vi "Teleop.vi"(10 "Match Info":T1={"Autonomous Elapsed Seconds"=0.0, "TeleOp Elapsed Seconds"=0.0, "Disabled Elapsed Seconds"=0.0, "Visited Autonomous"=FALSE, "Visited TeleOp"=FALSE, "Visited Disabled"=FALSE, "Autonomous Settings"={"Autonomous Style"=enum."Independent", "VI Refnum"=refnum}}, 11 "Call Context":T2) -> ()   [LabVIEW 2015]
doc: "This VI is called for each TeleOp packet received from the DS where the robot is not disabled. It is often used to read from the joysticks and update I/O or to update setpoints for timed control loops. It should complete and return within 20 milliseconds or it may miss DS packets."
uses:
  <vilib>/Rock Robotics/WPI/DriverStation/WPI_DriverStationDerivedRobotMode.ctl
  <vilib>/Rock Robotics/WPI/DriverStation/WPI_DriverStationMatch Info.ctl
  Refname/Refname Enum (Joystick).ctl
  Typedefs/Logitech Axis Mapping.ctl
  Action/Action Name.ctl
  Refname/Refname to String (Joystick).vi
  <vilib>/Rock Robotics/WPI/Utilities/WPI_GetSetVariantRefNum.vi
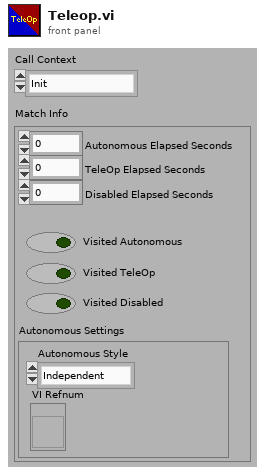
[diagram p1: front panel]
types:
  T1 = typedef "WPI_DriverStationMatch Info.ctl" = cluster{"Autonomous Elapsed Seconds":dbl, "TeleOp Elapsed Seconds":dbl, "Disabled Elapsed Seconds":dbl, "Visited Autonomous":bool, "Visited TeleOp":bool, "Visited Disabled":bool, "Autonomous Settings":cluster{"Autonomous Style":enum16{"Iterative", "Independent"}, "VI Refnum":refnum<vi>}}
  T2 = typedef "WPI_DriverStationDerivedRobotMode.ctl" = enum16{"Init", "Execute", "Stop"}
  T3 = typedef "Refname Enum (Joystick).ctl" = enum16{"Joystick 0", "Joystick 1", "Joystick 2", "Joystick 3"}
  T4 = typedef "WPI_JoystickDevRef.ctl" = cluster{"Device":T5}
  T5 = typedef "WPI_JoystickDeviceEnum.ctl" = enum16{"USB 0", "USB 1", "USB 2", "USB 3", "USB 4", "USB 5"}
  T6 = typedef "Logitech Axis Mapping.ctl" = enum32{"Left X Axis", "Left Y Axis", "Right X Axis", "Right Y Axis"}
  T7 = typedef "Action Name.ctl" = enum16{"No Action", "Drive Left", "Drive Right"}
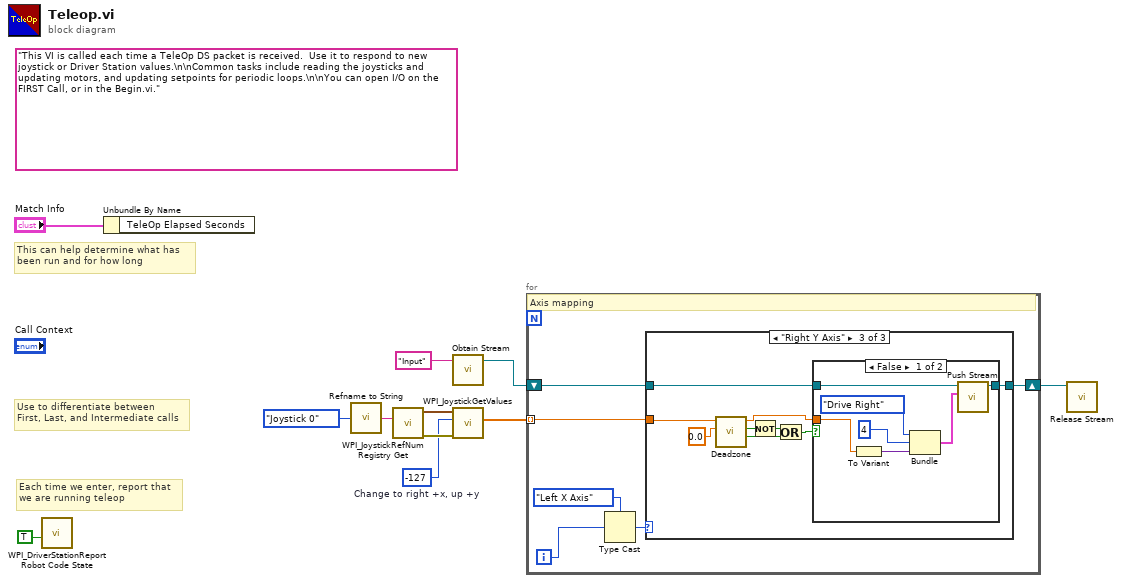
[diagram p0: block diagram]
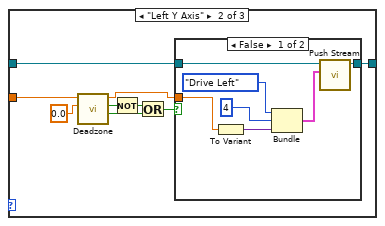
[diagram p3: hidden frame]
diagram:
  w4 = i8 -127  # Change to right +x, up +y
  (unwired) "This VI is called each time a TeleOp DS packet is received.  Use it to respond to new joystick or Driver Station values.\n\nCommon tasks include reading the joysticks and updating motors, and updating setpoints for periodic loops.\n\nYou can open I/O on the FIRST Call, or in the Begin.vi."
  # "Each time we enter, report that\nwe are running teleop"
  # "Use to differentiate between\nFirst, Last, and Intermediate calls"
  # "This can help determine what has\nbeen run and for how long"
  n1 = call <vilib>:"WPI_DriverStationReport Robot Code State.vi"("TeleOp"=TRUE ("Autonomous")) -> ()  [unwired: 10 in, 1 out]
  n2 = Unbundle By Name("Match Info") -> ()  [unwired: 1 out]
  n3 = call-poly "Refname to String.vi"("Joystick Refname"=Refname_Enum_(Joystick)."Joystick 0") -> ("Refnum Name"=w8:string)
  n4 = call <vilib>:"WPI_JoystickRefNum Registry Get.vi"("refnum name"=w8) -> ("error out"=w6:errorcluster, "JoystickDevRef"=w5:T4)  [unwired: 9 in]
  n5 = call "Obtain Stream.vi"("Name"="Input") -> ("stream out"=w2:refnum<queue>)  [unwired: 9 in, 1 out]
  n6 = call <vilib>:"WPI_JoystickGetValues.vi"("error in (no error)"=w6, "Scaler"=w4, "JoystickDevRef"=w5) -> ("Axes"=w3:dbl[])  [unwired: 4 in, 4 out]
  n7 = for {
    tunnel: w3 -> [w14] mode=indexing
    shift-right: [w12] -> w1
    shift-left: w2 -> [w13]
    i -> [w16]
    # "Axis mapping"
    n8 = Type Cast(type=Logitech_Axis_Mapping."Left X Axis" ("Axis Mapping"), x=w16) -> (*(type *) &x=w15:T6)
    n9 = case shown="\"Right Y Axis\"" w15 {
      tunnel: w14 -> [_ w23 w38]
      tunnel: w13 -> [w18 w20 w37]
      tunnel: [w18 w19 w36] -> w12
      frame Default {
      }
      frame "Left Y Axis" {
        n10 = call "Deadzone.vi"("Deadzone"=0.0, "Input"=w23) -> ("Just entered deadzone?"=w22:bool, "In deadzone?"=w26:bool, "Output"=w21:dbl)  [unwired: 6 in, 1 out]
        n11 = Not(x=w26) -> (.not. x?=w25:bool)
        n12 = Or(x=w25, y=w22) -> (x .or. y?=w27:bool)
        n13 = case shown="False" w27 {
          tunnel: w21 -> [w33 _]
          tunnel: w20 -> [w29 w35]
          tunnel: [w28 w35] -> w19
          frame False {
            n14 = To Variant(anything=w33) -> (Variant=w34:variant)
            n15 = Bundle("Name"=Action_Name."Drive Left", 4, "Variant"=w34) -> (w30:cluster{"Name":T7, i32, "Variant":variant})  [unwired: 1 in]
            n16 = call "Push Stream.vi"("action"=w30, "stream in"=w29) -> ("stream out"=w28:refnum<queue>)  [unwired: 8 in, 1 out]
          }
          frame True {
          }
        }
      }
      frame "Right Y Axis" {
        n17 = call "Deadzone.vi"("Deadzone"=0.0, "Input"=w38) -> ("Just entered deadzone?"=w40:bool, "In deadzone?"=w43:bool, "Output"=w39:dbl)  [unwired: 6 in, 1 out]
        n18 = Not(x=w43) -> (.not. x?=w42:bool)
        n19 = Or(x=w42, y=w40) -> (x .or. y?=w44:bool)
        n20 = case shown="False" w44 {
          tunnel: w39 -> [w50 _]
          tunnel: w37 -> [w46 w52]
          tunnel: [w45 w52] -> w36
          frame False {
            n21 = To Variant(anything=w50) -> (Variant=w51:variant)
            n22 = Bundle("Name"=Action_Name."Drive Right", 4, "Variant"=w51) -> (w47:cluster{"Name":T7, i32, "Variant":variant})  [unwired: 1 in]
            n23 = call "Push Stream.vi"("action"=w47, "stream in"=w46) -> ("stream out"=w45:refnum<queue>)  [unwired: 8 in, 1 out]
          }
          frame True {
          }
        }
      }
    }
  }
  n24 = call "Release Stream.vi"("stream in"=w1) -> ()  [unwired: 9 in, 2 out]
